vi "Set Iteration Count.vi"(8 "error in (no error)":errorcluster, 10 "iteration":u64=1, 11 "Timing in":refnum<class "Engine Timing.lvclass">) -> (0 "error out":errorcluster, 3 "Timing out":refnum<class "Engine Timing.lvclass">)   [LabVIEW 2017, in "Data Sharing Framework Core.lvlib" / "Data Sharing Framework Engine.lvlib" / "Engine Timing.lvclass"]
uses:
  Engine Timing.lvclass
  Engine Timing.lvclass/Engine Timing.ctl
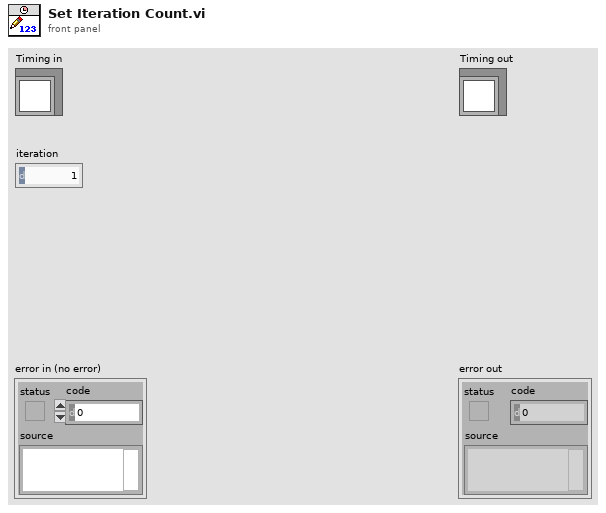
[diagram p1: front panel]
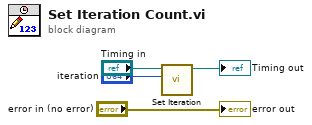
[diagram p0: block diagram]
diagram:
  n1 = call "Set Iteration.vi"("Iteration"="iteration", "Timing in"="Timing in") -> ("Timing out"=→"Timing out":refnum<class "Engine Timing.lvclass">)  [unwired: 9 in]
  "error out" <- "error in (no error)"
